vi "Set Label.vi"(8 "error in (no error)":errorcluster, 10 "Label":string, 11 "Search in":refnum<class "Search.lvclass">) -> (0 "error out":errorcluster, 3 "Search out":refnum<class "Search.lvclass">)   [LabVIEW 2016, in "Better Search.lvlib" / "Search.lvclass"]
uses:
  Search.lvclass
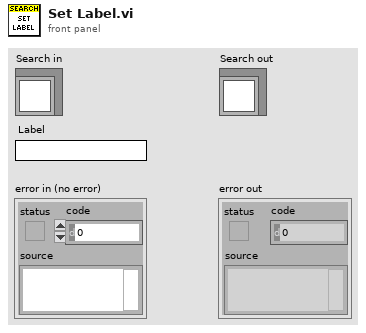
[diagram p1: front panel]
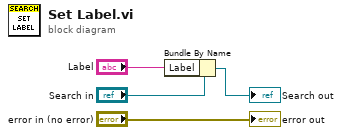
[diagram p0: block diagram]
diagram:
  n1 = Bundle By Name(cluster="Search in", "Label"="Label") -> (→"Search out":refnum<class "Search.lvclass">)
  "error out" <- "error in (no error)"
